vi "tdms.parse_properties.vi"(10 "Property Values":variant[](array[variant]), 11 "Property Names":string[](array[string])) -> (3 "Property Map":map{string, string}(c390))   [LabVIEW 2020, in "Nominal Client.lvclass"]
uses:
  Nominal Client.lvclass
  da61fce3-8bfd-4459-b653-c10878d9ea22.vi
  <vilib>/LabVIEW Open Source Project/Epoch Date & Time/formatter.iso8601/Timestamp to ISO8601 UTC DateTime.vi
  Nominal Client.lvclass/Nominal Client.ctl
  <vilib>/Utility/Data Type/NI_Data Type.lvlib
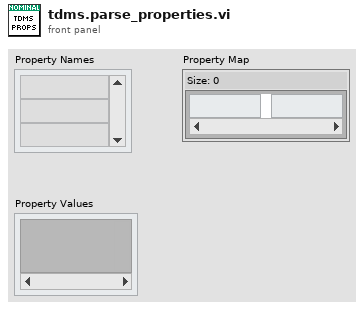
[diagram p1: front panel]
types:
  T1 = typedef "NI_Data Type.lvlib/Data Type.ctl" = enum8{"Invalid Type", "Void", "I8", "I16", "I32", "I64", "U8", "U16", "U32", "U64", "Single Float", "Double Float", "Extended Float", "Single Complex", "Double Complex", "Extended Complex", "Enum U8", "Enum U16", "Enum U32", "Enum U64", "Single Float With Unit", "Double Float With Unit", "Extended Float With Unit", "Single Complex with Unit", "Double Complex with Unit", "Extended Complex with Unit", "Boolean", "String", "Path", "Picture", "Tag", "Array", "Cluster", "Variant", "LV Variant", "Waveform", "Timestamp", "Digital Waveform", "Digital Data", "ExpressData", "Refnum", "External Data", "VI", "Poly VI", "LabVIEW Class Instance", "Fixed Point", "Set Collection", "Map Collection"}
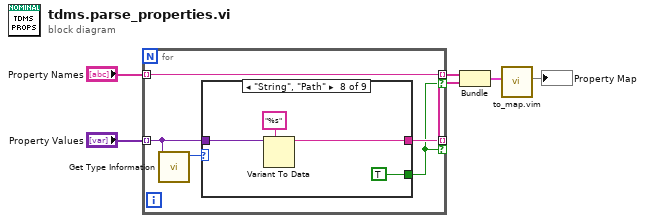
[diagram p0: block diagram]
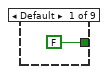
[diagram p2: hidden frame]
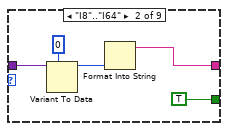
[diagram p3: hidden frame]
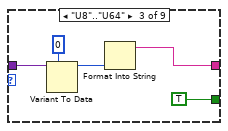
[diagram p4: hidden frame]
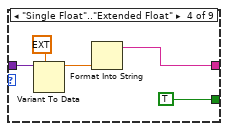
[diagram p5: hidden frame]
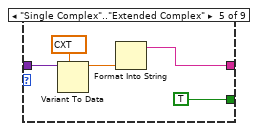
[diagram p6: hidden frame]
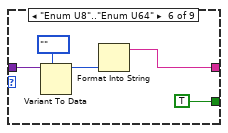
[diagram p7: hidden frame]
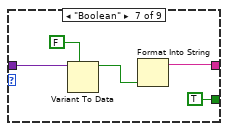
[diagram p8: hidden frame]
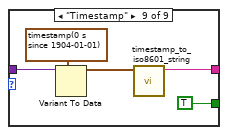
[diagram p9: hidden frame]
diagram:
  n1 = for {
    tunnel: "Property Values" -> [w10] mode=indexing
    tunnel: [w9] -> w6 mode=indexing if=w7
    tunnel: "Property Names" -> [w8] mode=indexing
    tunnel: [w8] -> w5 mode=indexing if=w7
    n2 = call <vilib>:"Get Type Information.vi"("variant"=w10) -> ("type"=w11:T1)  [unwired: 6 in, 4 out]
    n3 = case shown="\"String\", \"Path\"" w11 {
      tunnel: w10 -> [_ w17 w22 w25 w30 w36 w42 w46 w51]
      tunnel: [_ w14 w19 w24 w29 w34 w38 w44 w47] -> w9
      tunnel: [FALSE TRUE TRUE TRUE TRUE TRUE TRUE TRUE TRUE] -> w7
      frame Default {
      }
      frame "I8".."I64" {
        n4 = Variant To Data(type=i64 0, Variant=w17) -> (data=w15:i64)  [unwired: 1 in, 1 out]
        n5 = Format Into String(w15) -> (resulting string=w14:string)  [unwired: 3 in, 1 out]
      }
      frame "U8".."U64" {
        n6 = Variant To Data(type=u64 0, Variant=w22) -> (data=w20:u64)  [unwired: 1 in, 1 out]
        n7 = Format Into String(w20) -> (resulting string=w19:string)  [unwired: 3 in, 1 out]
      }
      frame "Single Float".."Extended Float" {
        n8 = Variant To Data(type=ext 0.0, Variant=w25) -> (data=w26:ext)  [unwired: 1 in, 1 out]
        n9 = Format Into String(w26) -> (resulting string=w24:string)  [unwired: 3 in, 1 out]
      }
      frame "Single Complex".."Extended Complex" {
        n10 = Variant To Data(type=cxt 0.0+0.0i, Variant=w30) -> (data=w31:cxt)  [unwired: 1 in, 1 out]
        n11 = Format Into String(w31) -> (resulting string=w29:string)  [unwired: 3 in, 1 out]
      }
      frame "Enum U8".."Enum U64" {
        n12 = Variant To Data(type=enum32{""}."", Variant=w36) -> (data=w37:enum32{""})  [unwired: 1 in, 1 out]
        n13 = Format Into String(w37) -> (resulting string=w34:string)  [unwired: 3 in, 1 out]
      }
      frame "Boolean" {
        n14 = Variant To Data(type=FALSE, Variant=w42) -> (data=w39:bool)  [unwired: 1 in, 1 out]
        n15 = Format Into String(w39) -> (resulting string=w38:string)  [unwired: 3 in, 1 out]
      }
      frame "String", "Path" {
        n16 = Variant To Data(type="%s", Variant=w46) -> (data=w44:string)  [unwired: 1 in, 1 out]
      }
      frame "Timestamp" {
        n17 = Variant To Data(type=timestamp(0 s since 1904-01-01), Variant=w51) -> (data=w48:timestamp)  [unwired: 1 in, 1 out]
        n18 = call "timestamp_to_iso8601_string.vi"("Time Stamp (now)"=w48) -> ("ISO8601 UTC DateTime"=w47:string)  [unwired: 10 in]
      }
    }
  }
  n19 = Bundle(w5, w6) -> (w4:cluster{string[], string[]})  [unwired: 1 in]
  n20 = call "to_map.vim"("Map"=w4) -> ("Map out"=→"Property Map":map{string, string})  [unwired: 10 in]
